vi "Main.vi"() -> ()   [LabVIEW 2024]
uses:
  <vilib>/userDefined/High Color/IMAQdx.ctl
  <vilib>/Utility/error.llb/DialogType.ctl
  <vilib>/addons/database/Connection.llb/Conn ObjectReference.ctl
  <vilib>/vision/Image Controls.llb/IMAQ Image.ctl
  <vilib>/vision/driver/IMAQdx.llb/IMAQdx Camera Control Mode.ctl
  <vilib>/addons/_JKI Toolkits/State Machine/_JKI_lib_State_Machine.llb/Select State(s)_err__jki_lib_state_machine.vi
  <vilib>/addons/_JKI Toolkits/State Machine/_JKI_lib_State_Machine.llb/Periodic Trigger__ogtk__JKI-SM__jki_lib_state_machine.vi
  <vilib>/addons/database/Auxilliary.llb/DB Tools Format Datetime String (Time Stamp).vi
  <vilib>/addons/database/NI_Database_API.lvlib
  <vilib>/vision/driver/NI_Vision_Acquisition_Software.lvlib
  <vilib>/addons/database/Connection.llb/DB Tools Open Connec (String).vi
panel:
  out "Error":bool
  out "Alarm":bool
  out "Measurement":dbl format="%#.2f"
  out "Database Save":bool
  out "Measuring":bool
  out "Is Measurement On":bool
  in  "Threshold":dbl(slide) min=0.0 max=100.0 step=5.0 scale=0.0..100.0
  in  "Source":bool
  in  "Camera":T1
  in  "Stop Application":bool
  in  "Stop Measurement":bool
  in  "Start Measurement":bool
  out "Image":T2(plugin-control)
  # "WLMS - Water Level Measuring\nSystem"
  # "Indicators"
  # "Is Measurement On"
  # "Currently Measuring"
  # "Saving To Database"
  # "Measurement Result, %"
  # "Alarm Level Detected"
  # "Error Occurred"
  # "Controls"
  # "Measurement Source"
  # "Camera"
  # "Image"
  # "Camera Source"
  # "Alarm Level Threshold"
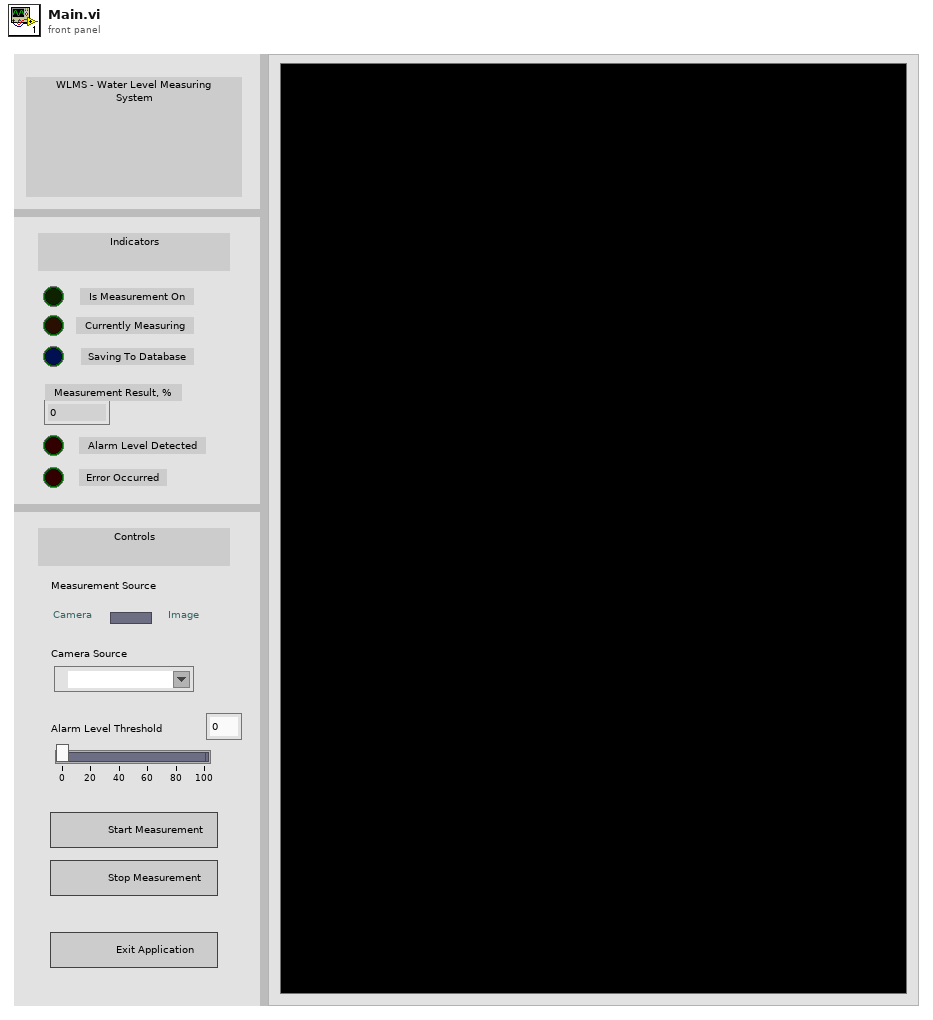
[diagram p1: front panel]
types:
  T1 = typedef "IMAQdx.ctl" = refnum<k21>
  T2 = typedef "IMAQ Image.ctl" = refnum<image>
  T3 = enum32{"Invalid", "Standard", "Closed", "Hidden", "Minimized", "Maximized"}
  T4 = enum32{"invalid app kind", "Development System", "Run Time System", "Student Edition", "Embedded LabVIEW", "Evaluation", "Custom"}
  T5 = typedef "NI_Vision_Acquisition_Software.lvlib/IMAQdx Camera Control Mode.ctl" = enum32{"Controller", "Listener"}
  T6 = typedef "NI_Database_API.lvlib/Conn ObjectReference.ctl" = refnum<k1>
  T7 = cluster{"Core":cluster{"Current VI Reference":refnum<vi>, "Close Panel on Exit?":bool}, "DB info":cluster{"DB connection":T6, "Table name":string, "Table columns":string[], "Connection string":string}, "Python info":cluster{"Function name":string, "Module name":string, "Python version":string, "Session reference":refnum<k35>}, "Measurement":cluster{"Is On":bool, "Period":u32, "Date":string, "Value":dbl, "Threshold":dbl, "Is Alarm On":bool, "LinePosY":i32}, "Camera data":cluster{"Camera":T1, "Image":T2, "Timeout":i32, "Frequency":i32, "Use image":bool, "Image name":string}}
  T8 = typedef "DialogType.ctl" = u16
  T9 = cluster{"Camera":T1, "Image":T2, "Timeout":i32, "Frequency":i32, "Use image":bool, "Image name":string}
  T10 = cluster{"Is On":bool, "Period":u32, "Date":string, "Value":dbl, "Threshold":dbl, "Is Alarm On":bool, "LinePosY":i32}
  T11 = cluster{"Function name":string, "Module name":string, "Python version":string, "Session reference":refnum<k35>}
  T12 = cluster{"DB connection":T6, "Table name":string, "Table columns":string[], "Connection string":string}
  T13 = cluster{"Current VI Reference":refnum<vi>, "Close Panel on Exit?":bool}
  T14 = cluster{"Desired Font (Application)":enum16{"User-specified Font", "Application Font", "System Font", "Dialog Font"}, "[User-specified Font]":cluster{"Font Name":string, "Size":i16, "Strikeout?":bool, "Italic?":bool, "Underline?":bool, "Outline?":bool, "Shadow?":bool, "Bold?":bool, "Rotation Angle":dbl}, "Horizontal Alignment":i16, "Vertical Alignment":i16}
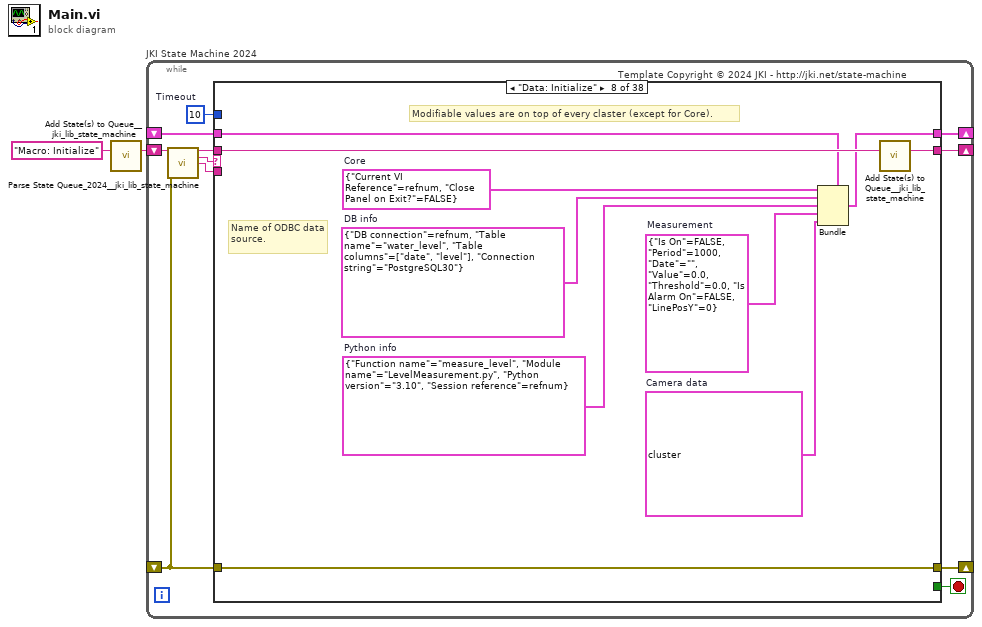
[diagram p0: block diagram]
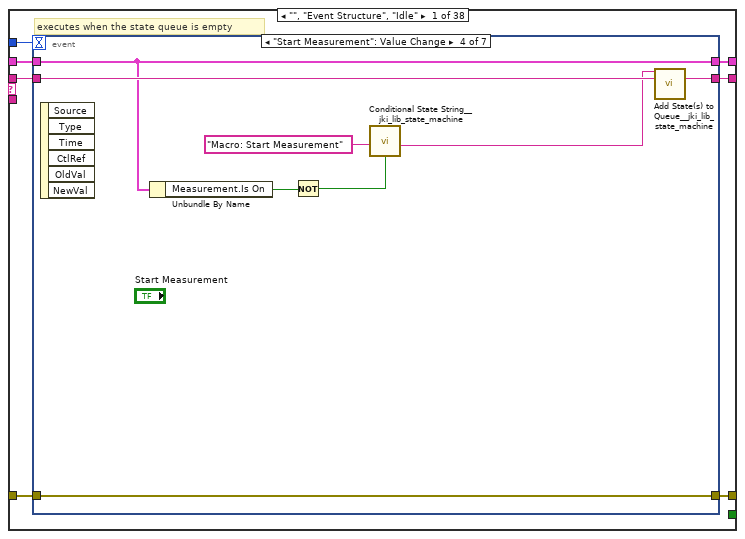
[diagram p2: hidden frame]
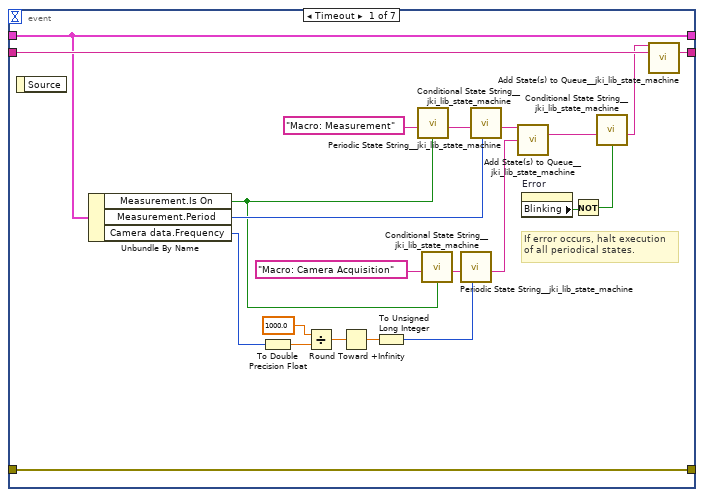
[diagram p3: hidden frame]
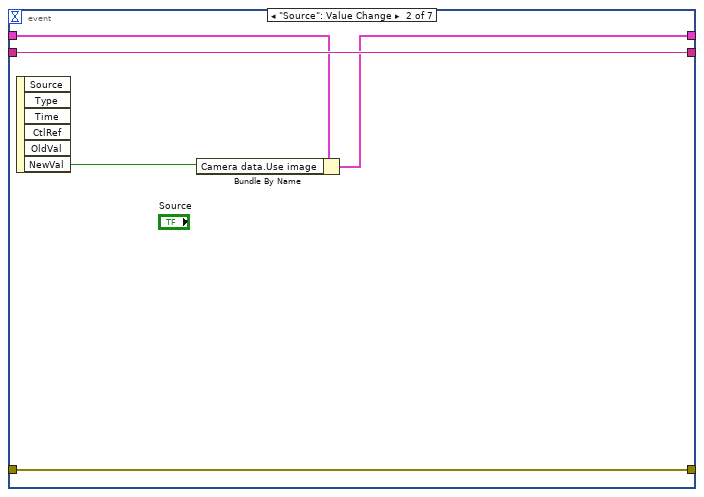
[diagram p4: hidden frame]
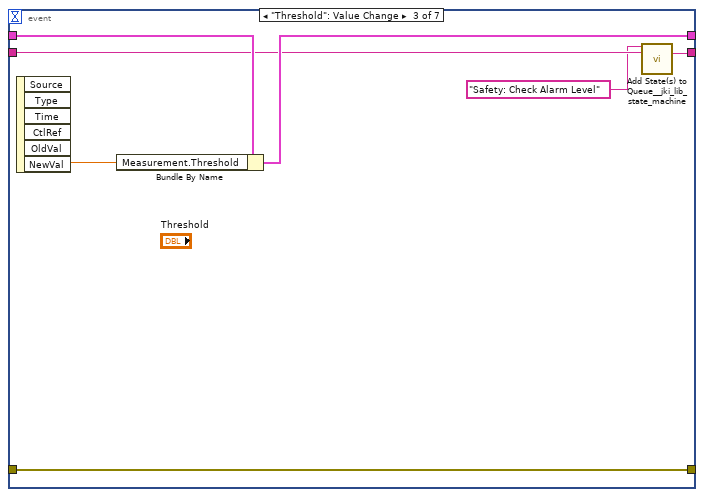
[diagram p5: hidden frame]
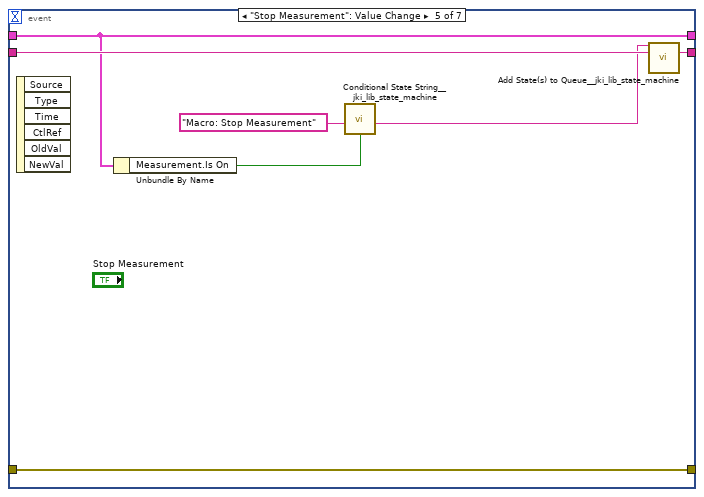
[diagram p6: hidden frame]
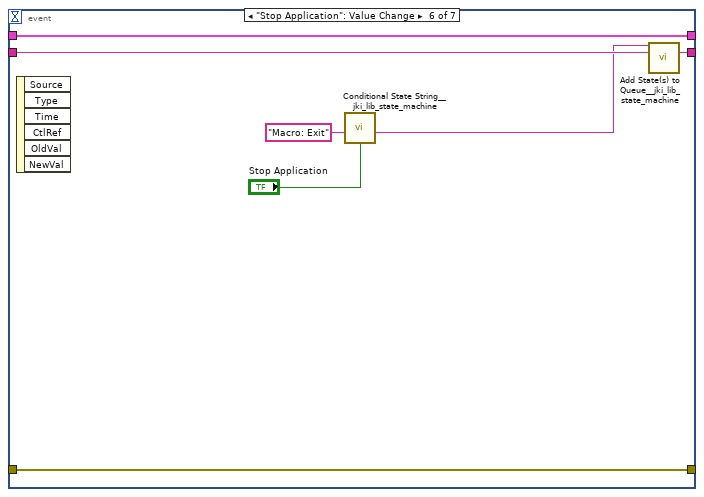
[diagram p7: hidden frame]
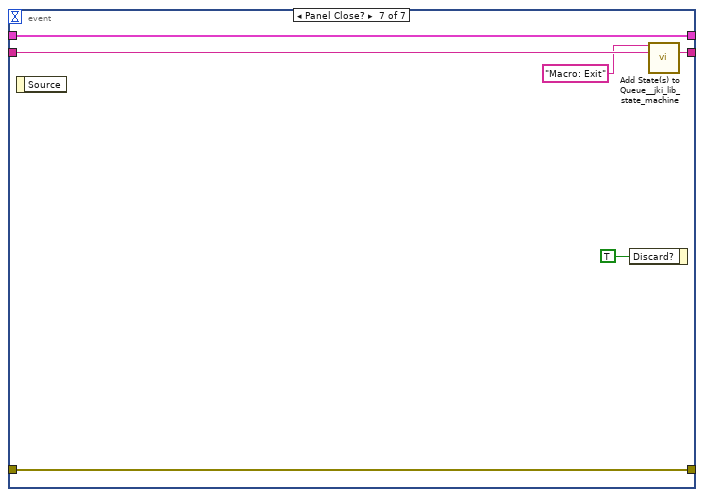
[diagram p8: hidden frame]
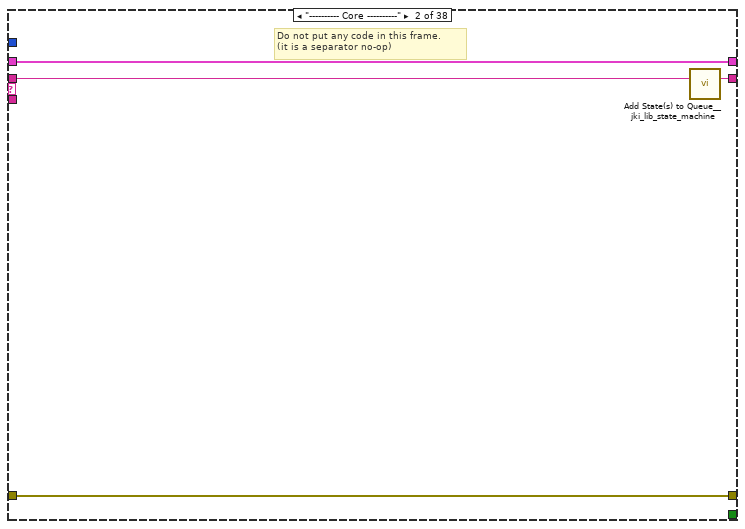
[diagram p9: hidden frame]
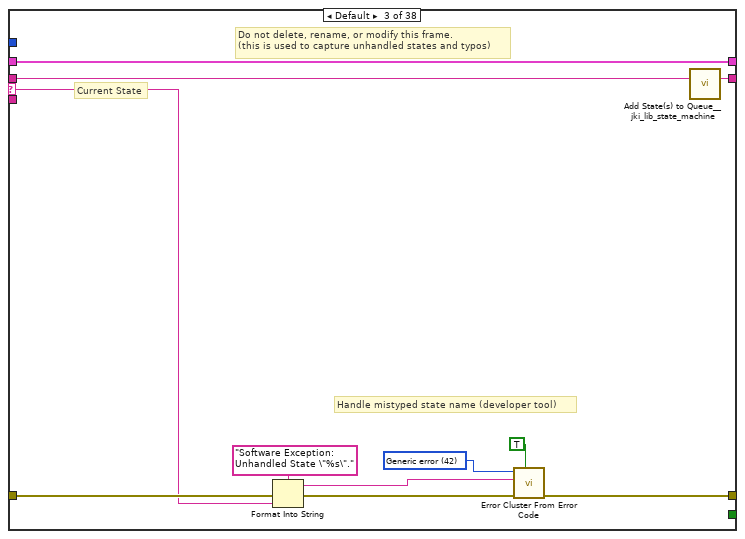
[diagram p10: hidden frame]
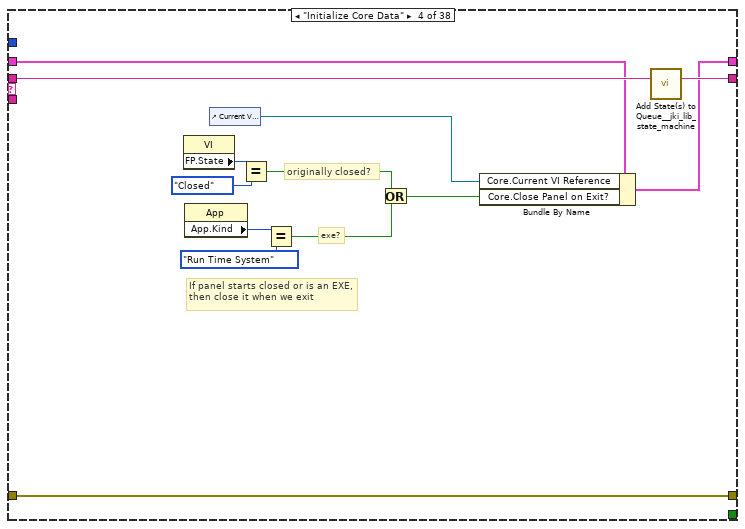
[diagram p11: hidden frame]
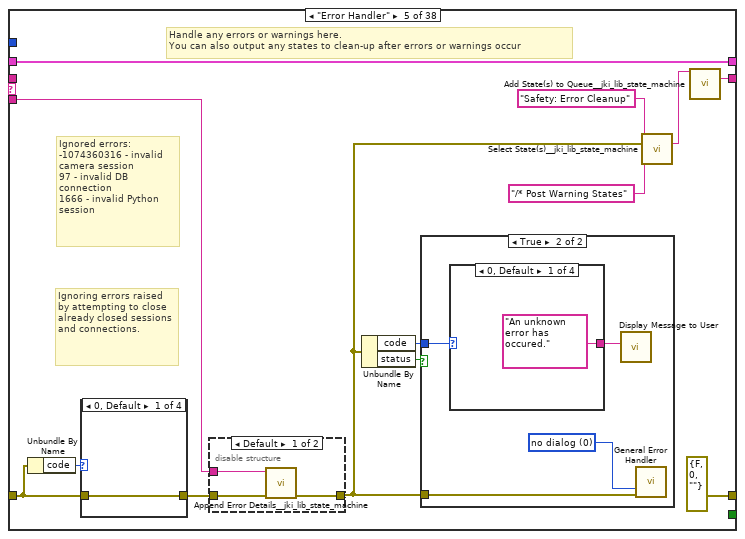
[diagram p12: hidden frame]
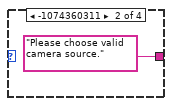
[diagram p14: hidden frame]
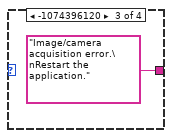
[diagram p15: hidden frame]
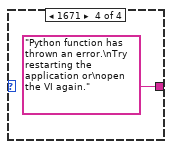
[diagram p16: hidden frame]
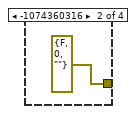
[diagram p17: hidden frame]
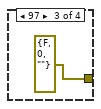
[diagram p18: hidden frame]
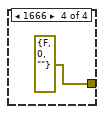
[diagram p19: hidden frame]
diagram:
  n1 = call <vilib>:"Add State(s) to Queue__jki_lib_state_machine.vi"("State(s) in (\"\")"="Macro: Initialize") -> ("States Out"=w2:string)  [unwired: 14 in]
  n2 = while "JKI State Machine 2024" {
    shift-right: [w7] -> _
    shift-left: _ -> [w6]
    shift-right: [w10] -> _
    shift-left: _ -> [w4]
    shift-right: [w9] -> _
    shift-left: w2 -> [w11]
    stop <- w8 stop-if-true
    w5 = 10  # Timeout
    # "Template Copyright © 2024 JKI - http://jki.net/state-machine"
    n3 = call <vilib>:"Parse State Queue_2024__jki_lib_state_machine.vi"("State Queue"=w11, "Error In (no error)"=w4) -> ("Remaining States"=w13:string, "Current State"=w3:string, "Arguments"=w12:string)  [unwired: 11 in]
    n4 = case shown="\"Data: Initialize\"" w3 {
      selector: w3 -> [_ _ w87 _ _ _ _ _ _ _ _ _ _ _ _ _ _ _ _ _ _ _ _ _ _ _ _ _ _ _ _ _ _ _ _ _ _ _]
      tunnel: w13 -> [w20 w86 w91 w110 _ w144 w148 w158 w164 w168 w179 w189 w195 w206 w270 w275 w283 w288 w295 w300 w312 w316 w324 w340 w346 w350 w364 w376 w421 w426 w432 w436 w444 w466 w472 w476 w485 w493]
      tunnel: w12 -> [_ _ _ _ w121 _ _ _ _ _ _ _ w190 w201 _ _ _ _ _ _ _ _ _ _ _ _ _ _ _ _ _ _ _ _ _ _ _ _]
      tunnel: w6 -> [w18 w83 w89 w98 w117 w142 w145 w149 w159 w165 w174 w181 w193 w200 w267 w272 w280 w284 w292 w297 w305 w313 w318 w333 w342 w347 w359 w374 w419 w422 w430 w433 w439 w456 w468 w473 w480 w488]
      tunnel: [w17 w84 w93 w108 errorcluster {"status"=FALSE, "code"=0, "source"=""} ("error out") w141 w146 w156 w161 w166 w177 w182 w191 w203 w268 w273 w278 w286 w290 w298 w308 w314 w319 w331 w343 w348 w351 w367 w399 w424 w427 w434 w440 w452 w469 w474 w483 w489] -> w10
      tunnel: w4 -> [w14 w84 w92 w108 w112 w141 w146 w156 w162 w166 w177 w183 w192 w204 w268 w273 w278 w286 w290 w298 w308 w314 w322 w337 w344 w348 w361 w371 w402 w424 w428 w434 w441 w464 w470 w474 w483 w489]
      tunnel: [w19 w85 w90 w109 w123 w143 w147 w157 w163 w167 w178 w188 w194 w205 w269 w274 w282 w287 w294 w299 w311 w315 w323 w339 w345 w349 w363 w375 w420 w425 w431 w435 w443 w465 w471 w475 w484 w492] -> w9
      tunnel: [_ _ _ _ _ TRUE _ _ _ _ _ _ _ _ _ _ _ _ _ _ _ _ _ _ _ _ _ _ _ _ _ _ _ _ _ _ _ _] -> w8
      tunnel: [w16 w83 w89 w99 w117 w142 w145 w152 w159 w165 w173 w181 w193 w200 w267 w272 w279 w284 w291 w297 w305 w313 w320 w333 w342 w347 w358 w373 w418 w422 w430 w433 w437 w455 w468 w473 w478 w487] -> w7
      tunnel: w5 -> [w15 _ _ _ _ _ _ _ _ _ _ _ _ _ _ _ _ _ _ _ _ _ _ _ _ _ _ _ _ _ _ _ _ _ _ _ _ _]
      frame "", "Event Structure", "Idle" {
        # "executes when the state queue is empty"
        n5 = event shown="[3] \"Start Measurement\": Value Change" {
          selector: _ -> [_ _ _ _ _ _ _]
          dyn-events: _ -> [_ _ _ _ _ _ _]
          timeout: w15 -> [_ _ _ _ _ _ _]
          tunnel: w20 -> [w42 w47 w49 w59 w69 w76 w82]
          tunnel: [w41 w47 w50 w60 w68 w75 w81] -> w19
          tunnel: w18 -> [w36 w46 w53 w57 w64 w73 w79]
          tunnel: [w40 w43 w54 w62 w67 w74 w80] -> w17
          tunnel: w14 -> [w40 w43 w54 w62 w67 w74 w80]
          tunnel: [w36 w44 w52 w57 w64 w73 w79] -> w16
          event Timeout {
            # "If error occurs, halt execution\nof all periodical states."
            n6 = event-data() -> ()  [unwired: 1 in, 1 out]
            n7 = Unbundle By Name(w36) -> ("Measurement.Is On"=w33:bool, "Measurement.Period"=w37:u32, "Camera data.Frequency"=w27:i32)
            n8 = To Double Precision Float(number=w27) -> (double precision float=w28:dbl)
            n9 = Divide(x=1000.0, y=w28) -> (x/y=w26:dbl)
            n10 = Round Toward +Infinity(x=w26) -> (ceil(x): smallest int >= x=w25:dbl)
            n11 = To Unsigned Long Integer(number=w25) -> (unsigned 32bit integer=w29:u32)
            n12 = call <vilib>:"Conditional State String__jki_lib_state_machine.vi"("Do State(s)?"=w33, "State"="Macro: Measurement") -> ("State Out"=w38:string)  [unwired: 7 in]
            n13 = call <vilib>:"Conditional State String__jki_lib_state_machine.vi"("Do State(s)?"=w33, "State"="Macro: Camera Acquisition") -> ("State Out"=w34:string)  [unwired: 7 in]
            n14 = call <vilib>:"Periodic State String__jki_lib_state_machine.vi"("Period (ms)"=w29, "State"=w34) -> ("State Out"=w31:string)  [unwired: 9 in]
            n15 = call <vilib>:"Periodic State String__jki_lib_state_machine.vi"("Period (ms)"=w37, "State"=w38) -> ("State Out"=w32:string)  [unwired: 9 in]
            n16 = call <vilib>:"Add State(s) to Queue__jki_lib_state_machine.vi"("State(s) in Front (\"\")"=w32, "State(s) at Back (\"\")"=w31) -> ("States Out"=w24:string)  [unwired: 13 in]
            n17 = property on="Error" class="Bool (strict)"() -> ("Blinking"=w22:bool)  [unwired: 2 in, 2 out]
            n18 = Not(x=w22) -> (.not. x?=w21:bool)
            n19 = call <vilib>:"Conditional State String__jki_lib_state_machine.vi"("Do State(s)?"=w21, "State"=w24) -> ("State Out"=w23:string)  [unwired: 7 in]
            n20 = call <vilib>:"Add State(s) to Queue__jki_lib_state_machine.vi"("State(s) in Front (\"\")"=w23, "State(s) in (\"\")"=w42) -> ("States Out"=w41:string)  [unwired: 13 in]
          }
          event "Source": Value Change {
            n21 = event-data() -> ("NewVal"=w45:bool)  [unwired: 1 in, 5 out]
            n22 = Bundle By Name(cluster=w46, "Camera data.Use image"=w45) -> (w44:T7)
          }
          event "Threshold": Value Change {
            n23 = event-data() -> ("NewVal"=w51:dbl)  [unwired: 1 in, 5 out]
            n24 = Bundle By Name(cluster=w53, "Measurement.Threshold"=w51) -> (w52:T7)
            n25 = call <vilib>:"Add State(s) to Queue__jki_lib_state_machine.vi"("State(s) in Front (\"\")"="Safety: Check Alarm Level", "State(s) in (\"\")"=w49) -> ("States Out"=w50:string)  [unwired: 13 in]
          }
          event "Start Measurement": Value Change {
            n26 = event-data() -> ()  [unwired: 1 in, 6 out]
            n27 = Unbundle By Name(w57) -> ("Measurement.Is On"=w56:bool)
            n28 = Not(x=w56) -> (.not. x?=w55:bool)
            n29 = call <vilib>:"Conditional State String__jki_lib_state_machine.vi"("Do State(s)?"=w55, "State"="Macro: Start Measurement") -> ("State Out"=w58:string)  [unwired: 7 in]
            n30 = call <vilib>:"Add State(s) to Queue__jki_lib_state_machine.vi"("State(s) in Front (\"\")"=w58, "State(s) in (\"\")"=w59) -> ("States Out"=w60:string)  [unwired: 13 in]
          }
          event "Stop Measurement": Value Change {
            n31 = event-data() -> ()  [unwired: 1 in, 6 out]
            n32 = Unbundle By Name(w64) -> ("Measurement.Is On"=w63:bool)
            n33 = call <vilib>:"Conditional State String__jki_lib_state_machine.vi"("Do State(s)?"=w63, "State"="Macro: Stop Measurement") -> ("State Out"=w65:string)  [unwired: 7 in]
            n34 = call <vilib>:"Add State(s) to Queue__jki_lib_state_machine.vi"("State(s) in Front (\"\")"=w65, "State(s) in (\"\")"=w69) -> ("States Out"=w68:string)  [unwired: 13 in]
          }
          event "Stop Application": Value Change {
            n35 = event-data() -> ()  [unwired: 1 in, 6 out]
            n36 = call <vilib>:"Conditional State String__jki_lib_state_machine.vi"("Do State(s)?"="Stop Application", "State"="Macro: Exit") -> ("State Out"=w71:string)  [unwired: 7 in]
            n37 = call <vilib>:"Add State(s) to Queue__jki_lib_state_machine.vi"("State(s) in Front (\"\")"=w71, "State(s) in (\"\")"=w76) -> ("States Out"=w75:string)  [unwired: 13 in]
          }
          event Panel Close? {
            n38 = event-data() -> ()  [unwired: 1 in, 1 out]
            n39 = event-data("Discard?"=TRUE) -> ()  [unwired: 1 in, 1 out]
            n40 = call <vilib>:"Add State(s) to Queue__jki_lib_state_machine.vi"("State(s) in Front (\"\")"="Macro: Exit", "State(s) in (\"\")"=w82) -> ("States Out"=w81:string)  [unwired: 13 in]
          }
        }
      }
      frame "---------- Core ----------" {
        # "Do not put any code in this frame.\n(it is a separator no-op)"
        n41 = call <vilib>:"Add State(s) to Queue__jki_lib_state_machine.vi"("State(s) in (\"\")"=w86) -> ("States Out"=w85:string)  [unwired: 14 in]
      }
      frame Default {
        w96 = 42 items=["No error", "Argument error", "Memory is full", "Out of zone", "End of file", "File already open", "Generic file I/O error", "File not found", "File permission error", "Disk is full", "Duplicate path", "Too many files open", "System feature not enabled", "Resource file not found", "Cannot add resource", "Resource not found", "Image not found", "Image memory error", "Pen does not exist", "Config type invalid", "Config token not found", "Config parse error", "Config memory error", "Bad external code format", "Bad external code offset", "External code not present", "Null window", "Destroy window error", "Null menu", "Print aborted", "Bad print record", "Print driver error", "Windows error during printing", "Memory error during printing", "Print dialog error", "Generic print error", "Invalid device refnum", "Device not found", "Device parameter error", "Device unit error", "Cannot open device", "Device call aborted", "Generic error", "Cancelled by user", "Object ID too low", "Object ID too high", "Object not in heap", "Unknown heap", "Unknown object (invalid DefProc)", "Unknown object (DefProc not in table)", "Message out of range", "Invalid (null) method", "Unknown message", "Manager call not supported", "Bad address", "Network operation in progress", "Network operation timed out", "Connection is busy", "Network attribute not supported", "Network error", "Address in use", "System out of memory", "Connection aborted", "Connection refused", "Not connected", "Already connected", "Connection closed", "Initialization error (interapplication manager)", "Bad occurrence", "Wait on unbound occurrence handler", "Occurrence queue overflow", "Datalog type conflict", "Unused", "Unrecognized type (interapplication manager)", "Memory corrupt", "Failed to make temporary DLL", "Old CIN version", "Drag socket not found", "Failed to load drop-object", "Failed to register OLE object", "Failed to release OLE object", "Format specifier type mismatch", "Unknown format specifier", "Too few format specifiers", "Too many format specifiers", "Scan failed", "Newer CIN version", "Error converting to variant", "Runtime menu error", "Password tampered", "Variant attribute not found", "Incompatible variant data type", "Event data is not available", "Event Store is not present", "Occurrence is not found", "Event Queue is not created", "Event info is not available", "Refnum passed is NULL", "Error retrieving Class GUID", "Error retrieving CoClass GUID", "Error retrieving TypeLib GUID.", "Bad built application magic bytes.", "Specific driver is different from the specific driver associated with the Logical Name.", "There is no session opened to the class driver.", "Max Error", "MAX - Error with config objects", "MAX - Error loading configuration", "MAX - Group not supported"]
        # "Current State"
        # "Do not delete, rename, or modify this frame.\n(this is used to capture unhandled states and typos)"
        # "Handle mistyped state name (developer tool)"
        n42 = Format Into String(format string="Software Exception: Unhandled State \"%s\"." ("message"), error in=w92, w87) -> (resulting string=w95:string, error out=w94:errorcluster)  [unwired: 1 in]
        n43 = call <vilib>:"Error Cluster From Error Code.vi"("show call chain? (False)"=TRUE, "error in (no error)"=w94, "error message (\"\")"=w95, "error code (0)"=w96) -> ("error out"=w93:errorcluster)  [unwired: 5 in]
        n44 = call <vilib>:"Add State(s) to Queue__jki_lib_state_machine.vi"("State(s) in (\"\")"=w91) -> ("States Out"=w90:string)  [unwired: 14 in]
      }
      frame "Initialize Core Data" {
        # "originally closed?"
        # "exe?"
        # "If panel starts closed or is an EXE, then close it when we exit"
        n45 = property class="VI"() -> ("FP.State"=w102:T3)  [unwired: 2 in, 2 out]
        n46 = property class="App"() -> ("App.Kind"=w107:T4)  [unwired: 2 in, 2 out]
        n47 = control-ref of="Current VI Reference"() -> (w103:refnum<vi>)
        n48 = Equal?(x=w102, y=T3."Closed" ("Front Panel Window:State")) -> (x = y?=w100:bool)
        n49 = Equal?(x=w107, y=T4."Run Time System" ("Application:Kind")) -> (x = y?=w105:bool)
        n50 = Or(x=w100, y=w105) -> (x .or. y?=w104:bool)
        n51 = Bundle By Name(cluster=w98, "Core.Current VI Reference"=w103, "Core.Close Panel on Exit?"=w104) -> (w99:T7)
        n52 = call <vilib>:"Add State(s) to Queue__jki_lib_state_machine.vi"("State(s) in (\"\")"=w110) -> ("States Out"=w109:string)  [unwired: 14 in]
      }
      frame "Error Handler" {
        # "Ignored errors:\n-1074360316 - invalid\ncamera session\n97 - invalid DB connection\n1666 - invalid Python session"
        # "Ignoring errors raised by attempting to close already closed sessions and connections."
        # "Handle any errors or warnings here.\nYou can also output any states to clean-up after errors or warnings occur"
        n53 = Unbundle By Name(w112) -> ("code"=w114:i32)
        n54 = case shown="0, Default" w114 {
          tunnel: [w132 errorcluster {"status"=FALSE, "code"=0, "source"=""} ("error out") errorcluster {"status"=FALSE, "code"=0, "source"=""} ("error out") errorcluster {"status"=FALSE, "code"=0, "source"=""} ("error out")] -> w113
          tunnel: w112 -> [w132 _ _ _]
          frame 0, Default {
          }
          frame -1074360316 {
          }
          frame 97 {
          }
          frame 1666 {
          }
        }
        n55 = disable-structure shown="Default" {
          disable-tunnel: w113 -> [w138 w139]
          disable-tunnel: w121 -> [w137 _]
          disable-tunnel: [w136 w139] -> w115
          frame condition #0 (active) {
            n56 = call <vilib>:"Append Error Details__jki_lib_state_machine.vi"("error in (no error)"=w138, "Previous State and Argument(s)"=w137) -> ("error out"=w136:errorcluster)  [unwired: 9 in]
          }
          frame condition #1 {
          }
        }
        n57 = Unbundle By Name(w115) -> ("code"=w116:i32, "status"=w111:bool)
        n58 = case shown="True" w111 {
          tunnel: w116 -> [_ w126]
          tunnel: w115 -> [_ w125]
          frame False {
          }
          frame True {
            w124 = T8 0 items=["no dialog", "OK message", "continue or stop message", "OK message + warnings", "continue/stop + warnings"] ("type of dialog (OK msg:1)")
            n59 = case shown="0, Default" w126 {
              tunnel: ["An unknown error has occured." "Please choose valid camera source." "Image/camera acquisition error.\nRestart the application." "Python function has thrown an error.\nTry restarting the application or\nopen the VI again."] -> w127
              frame 0, Default {
              }
              frame -1074360311 {
              }
              frame -1074396120 {
              }
              frame 1671 {
              }
            }
            n60 = call "Display Message to User"("Message"=w127) -> ()  [unwired: 9 in, 2 out]
            n61 = call <vilib>:"General Error Handler.vi"("type of dialog (OK msg:1)"=w124, "error in (no error)"=w125) -> ()  [unwired: 9 in, 5 out]
          }
        }
        n62 = call-poly <vilib>:"Select State(s)__jki_lib_state_machine.vi"("State(s) if True (\"\")"="Safety: Error Cleanup", "Select"=w115, "State(s) if False (\"\")"="/* Post Warning States") -> ("States Out"=w119:string)  [unwired: 12 in]
        n63 = call <vilib>:"Add State(s) to Queue__jki_lib_state_machine.vi"("State(s) in Front (\"\")"=w119) -> ("States Out"=w123:string)  [unwired: 14 in]
      }
      frame "Exit" {
        # "Do not put any code in this frame.\n(No errors that occur here will be handled.)"
        n64 = call <vilib>:"Add State(s) to Queue__jki_lib_state_machine.vi"("State(s) in (\"\")"=w144) -> ("States Out"=w143:string)  [unwired: 14 in]
      }
      frame "---------- Data ----------" {
        # "Do not put any code in this frame.\n(It is a separator no-op. You can make a copy of this frame to create a new Data frame)"
        n65 = call <vilib>:"Add State(s) to Queue__jki_lib_state_machine.vi"("State(s) in (\"\")"=w148) -> ("States Out"=w147:string)  [unwired: 14 in]
      }
      frame "Data: Initialize" {
        w150 = T9 {"Camera"="", "Image"=refnum, "Timeout"=5000, "Frequency"=25, "Use image"=TRUE, "Image name"="firstframe.jpg"}  # Camera data
        w151 = T10 {"Is On"=FALSE, "Period"=1000, "Date"="", "Value"=0.0, "Threshold"=0.0, "Is Alarm On"=FALSE, "LinePosY"=0}  # Measurement
        w153 = T11 {"Function name"="measure_level", "Module name"="LevelMeasurement.py", "Python version"="3.10", "Session reference"=refnum}  # Python info
        w154 = T12 {"DB connection"=refnum, "Table name"="water_level", "Table columns"=["date", "level"], "Connection string"="PostgreSQL30"}  # DB info
        w155 = T13 {"Current VI Reference"=refnum, "Close Panel on Exit?"=FALSE}  # Core
        # "Modifiable values are on top of every claster (except for Core)."
        # "Name of ODBC data source."
        n66 = Bundle(cluster=w149, "Core"=w155, "DB info"=w154, "Python info"=w153, "Measurement"=w151, "Camera data"=w150) -> (w152:T7)
        n67 = call <vilib>:"Add State(s) to Queue__jki_lib_state_machine.vi"("State(s) in (\"\")"=w158) -> ("States Out"=w157:string)  [unwired: 14 in]
      }
      frame "Data: Cleanup" {
        n68 = Unbundle By Name(w159) -> ("Core.Current VI Reference"=w160:refnum<vi>)
        n69 = Close Reference(reference=w160, error in (no error)=w162) -> (error out=w161:errorcluster)
        n70 = call <vilib>:"Add State(s) to Queue__jki_lib_state_machine.vi"("State(s) in (\"\")"=w164) -> ("States Out"=w163:string)  [unwired: 14 in]
      }
      frame "---------- UI ----------" {
        # "Do not put any code in this frame.\n(It is a separator no-op. You can make a copy of this frame to create a new UI frame)"
        n71 = call <vilib>:"Add State(s) to Queue__jki_lib_state_machine.vi"("State(s) in (\"\")"=w168) -> ("States Out"=w167:string)  [unwired: 14 in]
      }
      frame "UI: Initialize" {
        w171 = FALSE ("Database Save")
        n72 = property on="Source" class="Bool (strict)"() -> ("Value"=w175:bool)  [unwired: 2 in, 2 out]
        n73 = property on="Threshold" class="Slide (strict)"() -> ("Value"=w172:dbl)  [unwired: 2 in, 2 out]
        n74 = Bundle By Name(cluster=w174, "Camera data.Use image"=w175, "Measurement.Threshold"=w172) -> (w173:T7)
        n75 = property on="Is Measurement On" class="Bool (strict)"("Value"=w171) -> ()  [unwired: 2 in, 2 out]
        n76 = property on="Database Save" class="Bool (strict)"("Value"=w171) -> ()  [unwired: 2 in, 2 out]
        n77 = property on="Measuring" class="Bool (strict)"("Value"=w171) -> ()  [unwired: 2 in, 2 out]
        n78 = property on="Measurement" class="DigNum (strict)"("Value"=0.0 ("Measurement")) -> ()  [unwired: 2 in, 2 out]
        n79 = property on="Alarm" class="Bool (strict)"("Blinking"=FALSE) -> ()  [unwired: 2 in, 2 out]
        n80 = property on="Error" class="Bool (strict)"("Blinking"=FALSE) -> ()  [unwired: 2 in, 2 out]
        n81 = call <vilib>:"Add State(s) to Queue__jki_lib_state_machine.vi"("State(s) in (\"\")"=w179) -> ("States Out"=w178:string)  [unwired: 14 in]
      }
      frame "UI: Uninitialize" {
        w187 = FALSE ("Database Save")
        w185 = T2 refnum  # Image
        n82 = To Variant(anything=w185) -> (Variant=w184:variant)
        n83 = property on="Measuring" class="Bool (strict)"("Value"=w187) -> ()  [unwired: 2 in, 2 out]
        n84 = property on="Is Measurement On" class="Bool (strict)"("Value"=w187) -> ()  [unwired: 2 in, 2 out]
        n85 = property on="Database Save" class="Bool (strict)"("Value"=w187) -> ()  [unwired: 2 in, 2 out]
        n86 = property on="Measurement" class="DigNum (strict)"("Value"=0.0 ("Measurement")) -> ()  [unwired: 2 in, 2 out]
        n87 = property on="Image" class="ImageControl"("Value"=w184) -> ()  [unwired: 2 in, 2 out]
        n88 = Unbundle By Name(w181) -> ("Camera data.Image"=w180:T2)
        n89 = call "IMAQ Dispose"("Image"=w180, "error in (no error)"=w183) -> ("error out"=w182:errorcluster)  [unwired: 4 in]
        n90 = call <vilib>:"Add State(s) to Queue__jki_lib_state_machine.vi"("State(s) in (\"\")"=w189) -> ("States Out"=w188:string)  [unwired: 14 in]
      }
      frame "UI: Cursor Set" {
        # "Argument"
        n91 = case shown="\"Busy\"" w190 {
          tunnel: w192 -> [w197 w199]
          tunnel: [w196 w198] -> w191
          frame "Idle", Default {
            n92 = call <vilib>:"Unset Busy.vi"("error in (no error)"=w197) -> ("error out"=w196:errorcluster)  [unwired: 10 in]
          }
          frame "Busy" {
            n93 = call <vilib>:"Set Busy.vi"("error in (no error)"=w199) -> ("error out"=w198:errorcluster)  [unwired: 9 in, 1 out]
          }
        }
        n94 = call <vilib>:"Add State(s) to Queue__jki_lib_state_machine.vi"("State(s) in (\"\")"=w195) -> ("States Out"=w194:string)  [unwired: 14 in]
      }
      frame "UI: Front Panel State" {
        # "Argument"
        n95 = Unbundle By Name(w200) -> ("Core.Current VI Reference"=w202:refnum<vi>)
        n96 = case shown="\"Open\", \"Standard\", Default" w201 {
          tunnel: w204 -> [w212 w225 w236 w248 w260]
          tunnel: [w213 w226 w237 w249 w261] -> w203
          tunnel: w202 -> [_ _ _ _ _]
          frame "Open", "Standard", Default {
            w207 = T3."Standard" ("State")
            n97 = property class="VI"(error in=w212) -> (reference out=w210:refnum<vi>, error out=w211:errorcluster, "FP.State"=w209:T3)  [unwired: 1 in]
            n98 = Not Equal?(x=w209, y=w207) -> (x != y?=w208:bool)
            n99 = case shown="True" w208 {
              tunnel: [w217 w219] -> w213
              tunnel: w211 -> [w216 w219]
              tunnel: w210 -> [w215 _]
              tunnel: w207 -> [w214 _]
              frame True {
                n100 = invoke class="VI" method="FP.Open"(reference=w215, error in=w216, "Activate"=TRUE, "State"=w214) -> (error out=w217:errorcluster)  [unwired: 1 in, 4 out]
              }
              frame False {
              }
            }
          }
          frame "Close", "Closed" {
            n101 = property class="VI"(error in=w225) -> (reference out=w223:refnum<vi>, error out=w224:errorcluster, "FP.State"=w221:T3)  [unwired: 1 in]
            n102 = Not Equal?(x=w221, y=T3."Closed" ("Front Panel Window:State")) -> (x != y?=w220:bool)
            n103 = case shown="True" w220 {
              tunnel: [w227 w230] -> w226
              tunnel: w224 -> [w227 w229]
              tunnel: w223 -> [_ w228]
              frame False {
              }
              frame True {
                n104 = invoke class="VI" method="FP.Close"(reference=w228, error in=w229) -> (error out=w230:errorcluster)  [unwired: 1 in, 2 out]
              }
            }
          }
          frame "Hidden", "Hide" {
            w231 = T3."Hidden" ("State")
            n105 = property class="VI"(error in=w236) -> (reference out=w234:refnum<vi>, error out=w235:errorcluster, "FP.State"=w233:T3)  [unwired: 1 in]
            n106 = Not Equal?(x=w233, y=w231) -> (x != y?=w232:bool)
            n107 = case shown="True" w232 {
              tunnel: [w241 w242] -> w237
              tunnel: w235 -> [w240 w242]
              tunnel: w234 -> [w239 _]
              tunnel: w231 -> [w238 _]
              frame True {
                n108 = invoke class="VI" method="FP.Open"(reference=w239, error in=w240, "State"=w238) -> (error out=w241:errorcluster)  [unwired: 2 in, 4 out]
              }
              frame False {
              }
            }
          }
          frame "Minimize", "Minimized" {
            w243 = T3."Minimized" ("State")
            n109 = property class="VI"(error in=w248) -> (reference out=w246:refnum<vi>, error out=w247:errorcluster, "FP.State"=w245:T3)  [unwired: 1 in]
            n110 = Not Equal?(x=w245, y=w243) -> (x != y?=w244:bool)
            n111 = case shown="True" w244 {
              tunnel: [w253 w254] -> w249
              tunnel: w247 -> [w252 w254]
              tunnel: w246 -> [w251 _]
              tunnel: w243 -> [w250 _]
              frame True {
                n112 = invoke class="VI" method="FP.Open"(reference=w251, error in=w252, "State"=w250) -> (error out=w253:errorcluster)  [unwired: 2 in, 4 out]
              }
              frame False {
              }
            }
          }
          frame "Maximize", "Maximized" {
            w255 = T3."Maximized" ("State")
            n113 = property class="VI"(error in=w260) -> (reference out=w258:refnum<vi>, error out=w259:errorcluster, "FP.State"=w257:T3)  [unwired: 1 in]
            n114 = Not Equal?(x=w257, y=w255) -> (x != y?=w256:bool)
            n115 = case shown="True" w256 {
              tunnel: [w265 w266] -> w261
              tunnel: w259 -> [w264 w266]
              tunnel: w258 -> [w263 _]
              tunnel: w255 -> [w262 _]
              frame True {
                n116 = invoke class="VI" method="FP.Open"(reference=w263, error in=w264, "State"=w262) -> (error out=w265:errorcluster)  [unwired: 2 in, 4 out]
              }
              frame False {
              }
            }
          }
        }
        n117 = call <vilib>:"Add State(s) to Queue__jki_lib_state_machine.vi"("State(s) in (\"\")"=w206) -> ("States Out"=w205:string)  [unwired: 14 in]
      }
      frame "---------- Macro ----------" {
        # "Do not put any code in this frame.\n(It is a separator no-op. You can make a copy of this frame to create a new Macro frame)"
        n118 = call <vilib>:"Add State(s) to Queue__jki_lib_state_machine.vi"("State(s) in (\"\")"=w270) -> ("States Out"=w269:string)  [unwired: 14 in]
      }
      frame "Macro: Initialize" {
        w271 = "Data: Initialize\nInitialize Core Data\nUI: Initialize\nUI: Front Panel State >> Open"  # Data: Initialize Initialize Core Data UI: Initialize UI: Front Panel State >> Open
        n119 = call <vilib>:"Add State(s) to Queue__jki_lib_state_machine.vi"("State(s) in Front (\"\")"=w271, "State(s) in (\"\")"=w275) -> ("States Out"=w274:string)  [unwired: 13 in]
      }
      frame "Macro: Start Measurement" {
        w277 = TRUE ("Measurement.Is On")
        n120 = property on="Error" class="Bool (strict)"("Blinking"=FALSE) -> ()  [unwired: 2 in, 2 out]
        n121 = Bundle By Name(cluster=w280, "Measurement.Is On"=w277) -> (w279:T7)
        n122 = property on="Is Measurement On" class="Bool (strict)"("Value"=w277) -> ()  [unwired: 2 in, 2 out]
        n123 = call <vilib>:"Add State(s) to Queue__jki_lib_state_machine.vi"("State(s) in Front (\"\")"="Camera: Initialize\nDatabase: Connect\nPython: Open Session", "State(s) in (\"\")"=w283) -> ("States Out"=w282:string)  [unwired: 13 in]
      }
      frame "Macro: Measurement" {
        n124 = call <vilib>:"Add State(s) to Queue__jki_lib_state_machine.vi"("State(s) in Front (\"\")"="Python: Fetch Level\nSafety: Check Alarm Level\nDatabase: Save Data" ("State(s) in Front (\"\")"), "State(s) in (\"\")"=w288) -> ("States Out"=w287:string)  [unwired: 13 in]
      }
      frame "Macro: Stop Measurement" {
        w289 = FALSE ("Measurement.Is On")
        n125 = Bundle By Name(cluster=w292, "Measurement.Is On"=w289) -> (w291:T7)
        n126 = property on="Is Measurement On" class="Bool (strict)"("Value"=w289) -> ()  [unwired: 2 in, 2 out]
        n127 = call <vilib>:"Add State(s) to Queue__jki_lib_state_machine.vi"("State(s) in Front (\"\")"="Camera: Remove\nDatabase: Disconnect \nPython: Close Session", "State(s) in (\"\")"=w295) -> ("States Out"=w294:string)  [unwired: 13 in]
      }
      frame "Macro: Camera Acquisition" {
        n128 = call <vilib>:"Add State(s) to Queue__jki_lib_state_machine.vi"("State(s) in Front (\"\")"="Camera: Read\nCamera: Add Data\nCamera: Display" ("State(s) in Front (\"\")"), "State(s) in (\"\")"=w300) -> ("States Out"=w299:string)  [unwired: 13 in]
      }
      frame "Macro: Exit" {
        n129 = Unbundle By Name(w305) -> ("Core.Close Panel on Exit?"=w306:bool, "Measurement.Is On"=w303:bool)
        n130 = call <vilib>:"Conditional State String__jki_lib_state_machine.vi"("Do State(s)?"=w306, "State"="UI: Front Panel State >> Close") -> ("State Out"=w304:string)  [unwired: 7 in]
        n131 = call <vilib>:"Conditional State String__jki_lib_state_machine.vi"("Do State(s)?"=w303, "State"="Macro: Stop Measurement") -> ("State Out"=w301:string)  [unwired: 7 in]
        n132 = call <vilib>:"Add State(s) to Queue__jki_lib_state_machine.vi"("State(s) in Front (\"\")"=w304, "State(s) in (\"\")"=w301, "State(s) at Back (\"\")"="UI: Uninitialize\nData: Cleanup\nExit") -> ("States Out"=w309:string)  [unwired: 12 in]
        n133 = call <vilib>:"Add State(s) to Queue__jki_lib_state_machine.vi"("State(s) in Front (\"\")"=w309, "State(s) in (\"\")"=w312) -> ("States Out"=w311:string)  [unwired: 13 in]
      }
      frame "---------- Database ----------" {
        # "Do not put any code in this frame.\n(It is a separator no-op. You can make a copy of this frame to create a new Macro frame)"
        n134 = call <vilib>:"Add State(s) to Queue__jki_lib_state_machine.vi"("State(s) in (\"\")"=w316) -> ("States Out"=w315:string)  [unwired: 14 in]
      }
      frame "Database: Connect" {
        n135 = Unbundle By Name(w318) -> ("DB info.Connection string"=w317:string)
        n136 = call-poly <vilib>:"DB Tools Open Connection.vi"("error in (no error)"=w322, "connection information"=w317) -> ("error out"=w319:errorcluster, "connection reference"=w321:T6)  [unwired: 6 in]
        n137 = Bundle By Name(cluster=w318, "DB info.DB connection"=w321) -> (w320:T7)
        n138 = call <vilib>:"Add State(s) to Queue__jki_lib_state_machine.vi"("State(s) in (\"\")"=w324) -> ("States Out"=w323:string)  [unwired: 14 in]
      }
      frame "Database: Save Data" {
        # "Jeżeli nie ma błędu, status przyjmuje wartość false. Jest to wykorzystane do sterowania kontrolką informującą o trwającym zapisie do bazy danych."
        n139 = Unbundle By Name(w333) -> ("Measurement.Date"=w326:string, "Measurement.Value"=w327:dbl, "DB info.DB connection"=w334:T6, "DB info.Table name"=w336:string, "DB info.Table columns"=w335:string[])
        n140 = Bundle(cluster=cluster{string, dbl} {"", 0.0}, w326, w327) -> (w328:cluster{string, dbl})
        n141 = To Variant(anything=w328) -> (Variant=w325:variant)
        n142 = call <vilib>:"DB Tools Insert Data.vi"("create table? (F)"=TRUE, "data"=w325, "error in (no error)"=w337, "columns"=w335, "table"=w336, "connection reference"=w334) -> ("error out"=w331:errorcluster)  [unwired: 4 in, 1 out]
        n143 = Unbundle By Name(w331) -> ("status"=w330:bool)
        n144 = property on="Database Save" class="Bool (strict)"("Value"=w330) -> ()  [unwired: 2 in, 2 out]
        n145 = call <vilib>:"Add State(s) to Queue__jki_lib_state_machine.vi"("State(s) in (\"\")"=w340) -> ("States Out"=w339:string)  [unwired: 14 in]
        "Database Save" <- TRUE ("Database Save")
      }
      frame "Database: Disconnect" {
        n146 = Unbundle By Name(w342) -> ("DB info.DB connection"=w341:T6)
        n147 = call <vilib>:"DB Tools Close Connection.vi"("error in (no error)"=w344, "connection reference"=w341) -> ("error out"=w343:errorcluster)  [unwired: 5 in]
        n148 = call <vilib>:"Add State(s) to Queue__jki_lib_state_machine.vi"("State(s) in (\"\")"=w346) -> ("States Out"=w345:string)  [unwired: 14 in]
      }
      frame "---------- Camera ----------" {
        # "Do not put any code in this frame.\n(It is a separator no-op. You can make a copy of this frame to create a new Macro frame)"
        n149 = call <vilib>:"Add State(s) to Queue__jki_lib_state_machine.vi"("State(s) in (\"\")"=w350) -> ("States Out"=w349:string)  [unwired: 14 in]
      }
      frame "Camera: Initialize" {
        n150 = call <vilib>:"IMAQdx Open Camera.vi"("Camera Control Mode"=IMAQdx_Camera_Control_Mode."Controller", "error in"=w361, "Session In"="Camera") -> ("error out"=w357:errorcluster, "Session Out"=w356:T1)  [unwired: 7 in]
        n151 = call <vilib>:"IMAQdx Configure Grab.vi"("error in"=w357, "Session In"=w356) -> ("error out"=w353:errorcluster, "Session Out"=w355:T1)  [unwired: 8 in]
        n152 = call "IMAQ Create"("Image Name"="Measurement", "error in (no error)"=w353) -> ("New Image"=w352:T2, "error out"=w351:errorcluster)  [unwired: 3 in]
        n153 = Bundle By Name(cluster=w359, "Camera data.Camera"=w355, "Camera data.Image"=w352) -> (w358:T7)
        n154 = call <vilib>:"Add State(s) to Queue__jki_lib_state_machine.vi"("State(s) in (\"\")"=w364) -> ("States Out"=w363:string)  [unwired: 14 in]
      }
      frame "Camera: Read" {
        n155 = Unbundle By Name(w374) -> ("Camera data.Use image"=w366:bool, "Camera data.Timeout"=w372:i32, "Camera data.Camera"=w369:T1, "Camera data.Image"=w370:T2, "Camera data.Image name"=w365:string)
        n156 = case shown="True" w366 {
          tunnel: w372 -> [w382 _]
          tunnel: w371 -> [w381 w385]
          tunnel: w370 -> [w377 w386]
          tunnel: w369 -> [w380 _]
          tunnel: [w379 w384] -> w367
          tunnel: [w378 w383] -> w368
          tunnel: w365 -> [_ w388]
          frame False {
            n157 = call <vilib>:"IMAQdx Grab2.vi"("Timeout (ms)"=w382, "error in"=w381, "Image In"=w377, "Session In"=w380) -> ("error out"=w379:errorcluster, "Image Out"=w378:T2)  [unwired: 4 in, 2 out]
          }
          frame True {
            n158 = Current VI's Path() -> (path=w389:path)
            n159 = Strip Path(path=w389) -> (stripped path=w390:path)  [unwired: 1 out]
            n160 = Build Path(base path=w390, name or relative path=w388) -> (appended path=w387:path)
            n161 = call "IMAQ ReadFile 2"("File Path"=w387, "error in (no error)"=w385, "Image"=w386) -> ("error out"=w384:errorcluster, "Image Out"=w383:T2)  [unwired: 4 in, 3 out]
          }
        }
        n162 = Bundle By Name(cluster=w374, "Camera data.Image"=w368) -> (w373:T7)
        n163 = call <vilib>:"Add State(s) to Queue__jki_lib_state_machine.vi"("State(s) in (\"\")"=w376) -> ("States Out"=w375:string)  [unwired: 14 in]
      }
      frame "Camera: Add Data" {
        n164 = Unbundle By Name(w419) -> ("Camera data.Image"=w391:T2, "Measurement.Value"=w409:dbl, "Measurement.LinePosY"=w397:i32, "Measurement.Is Alarm On"=w396:bool)
        n165 = call "GetLinePoints.vi"("error in (no error)"=w402, "LinePosY"=w397, "Image"=w391) -> ("error out"=w403:errorcluster, "End Point"=w408:cluster{"X":i32, "Y":i32}, "Start Point"=w412:cluster{"X":i32, "Y":i32})  [unwired: 6 in]
        n166 = call "IMAQ Overlay Line"("Color"=u32 8388608, "error in (no error)"=w403, "End Point"=w408, "Start Point"=w412, "Image"=w391) -> ("error out"=w410:errorcluster, "Image Out"=w413:T2)  [unwired: 5 in]
        n167 = call "GetTextPoint.vi"("End Point"=w408, "Y Offset"=0 ("y"), "X Offset"=-20 ("y")) -> ("Text Point"=w414:cluster{"X":i32, "Y":i32})  [unwired: 8 in]
        n168 = call "TextProperties.vi"("Font Multiplier"=0.05 ("x"), "Image"=w391) -> ("error out"=w398:errorcluster, "Font, Size & Style"=w400:T14)  [unwired: 8 in]
        n169 = Select(t=u32 16711680 ("Text Color (black)"), s=w396, f=u32 0 ("Text Color (black)")) -> (s? t:f=w404:u32)
        n170 = call "FormatPercentage.vi"("Precision"=i16 2 ("precision (6)"), "Raw Percentage"=w409) -> ("Formatted Percentage"=w411:string)  [unwired: 9 in]
        n171 = call "IMAQ Overlay Text"("Text Color (black)"=w404, "Font, Size & Style"=w400, "error in (no error)"=w410, "String"=w411, "Origin"=w414, "Image"=w413) -> ("error out"=w394:errorcluster, "Image Out"=w393:T2)  [unwired: 4 in]
        n172 = call "IMAQ Merge Overlay"("error in (no error)"=w394, "Image Src"=w393) -> ("error out"=w395:errorcluster, "Image Dst Out"=w392:T2)  [unwired: 8 in]
        n173 = Merge Errors(w398, w395) -> (w399:errorcluster)
        n174 = Bundle By Name(cluster=w419, "Camera data.Image"=w392) -> (w418:T7)
        n175 = call <vilib>:"Add State(s) to Queue__jki_lib_state_machine.vi"("State(s) in (\"\")"=w421) -> ("States Out"=w420:string)  [unwired: 14 in]
      }
      frame "Camera: Display" {
        n176 = Unbundle By Name(w422) -> ("Camera data.Image"=→"Image":T2)
        n177 = call <vilib>:"Add State(s) to Queue__jki_lib_state_machine.vi"("State(s) in (\"\")"=w426) -> ("States Out"=w425:string)  [unwired: 14 in]
      }
      frame "Camera: Remove" {
        n178 = Unbundle By Name(w430) -> ("Camera data.Camera"=w429:T1)
        n179 = call <vilib>:"IMAQdx Close Camera.vi"("error in"=w428, "Session In"=w429) -> ("error out"=w427:errorcluster)  [unwired: 9 in]
        n180 = call <vilib>:"Add State(s) to Queue__jki_lib_state_machine.vi"("State(s) in (\"\")"=w432) -> ("States Out"=w431:string)  [unwired: 14 in]
      }
      frame "---------- Python ----------" {
        # "Do not put any code in this frame.\n(It is a separator no-op. You can make a copy of this frame to create a new Macro frame)"
        n181 = call <vilib>:"Add State(s) to Queue__jki_lib_state_machine.vi"("State(s) in (\"\")"=w436) -> ("States Out"=w435:string)  [unwired: 14 in]
      }
      frame "Python: Open Session" {
        n182 = Unbundle By Name(w439) -> ("Python info.Python version"=w442:string)
        n183 = Open Python Session(python version=w442, 3:w441) -> (session out=w438:refnum<k35>, error out=w440:errorcluster)  [unwired: 1 in]
        n184 = Bundle By Name(cluster=w439, "Python info.Session reference"=w438) -> (w437:T7)
        n185 = call <vilib>:"Add State(s) to Queue__jki_lib_state_machine.vi"("State(s) in (\"\")"=w444) -> ("States Out"=w443:string)  [unwired: 14 in]
      }
      frame "Python: Fetch Level" {
        # "If there's no error, the status is false, therefore we can say the measurement is done."
        n186 = Unbundle By Name(w456) -> ("Python info.Session reference"=w463:refnum<k35>, "Python info.Module name"=w460:string, "Python info.Function name"=w458:string, "Camera data.Use image"=w450:bool, "Camera data.Image name"=w449:string)
        n187 = Current VI's Path() -> (path=w462:path)
        n188 = Strip Path(path=w462) -> (stripped path=w461:path)  [unwired: 1 out]
        n189 = Build Path(base path=w461, name or relative path=w460) -> (appended path=w459:path)
        n190 = node(w463, w459, w458, w464, cluster{"Value":dbl, "LinePosY":i32} {"Value"=0.0, "LinePosY"=0}, w450, w449) -> (w452:errorcluster, w447:cluster{"Value":dbl, "LinePosY":i32})  [unwired: 2 in, 3 out]
        n191 = Get Date/Time In Seconds() -> (seconds since 1Jan1904=w457:timestamp)
        n192 = Unbundle By Name(w447) -> ("Value"=w445:dbl, "LinePosY"=w446:i32)
        "Measurement" <- w445
        n193 = call-poly <vilib>:"DB Tools Format Datetime String.vi"("time stamp"=w457) -> ("date/time string"=w454:string)
        n194 = Bundle By Name(cluster=w456, "Measurement.Date"=w454, "Measurement.Value"=w445, "Measurement.LinePosY"=w446) -> (w455:T7)
        n195 = Unbundle By Name(w452) -> ("status"=w451:bool)
        n196 = property on="Measuring" class="Bool (strict)"("Value"=w451) -> ()  [unwired: 2 in, 2 out]
        n197 = call <vilib>:"Add State(s) to Queue__jki_lib_state_machine.vi"("State(s) in (\"\")"=w466) -> ("States Out"=w465:string)  [unwired: 14 in]
        "Measuring" <- TRUE ("Measuring")
      }
      frame "Python: Close Session" {
        n198 = Unbundle By Name(w468) -> ("Python info.Session reference"=w467:refnum<k35>)
        n199 = Close Python Session(session in=w467, error in=w470) -> (11:w469:errorcluster)
        n200 = call <vilib>:"Add State(s) to Queue__jki_lib_state_machine.vi"("State(s) in (\"\")"=w472) -> ("States Out"=w471:string)  [unwired: 14 in]
      }
      frame "---------- Safety ----------" {
        # "Do not put any code in this frame.\n(It is a separator no-op. You can make a copy of this frame to create a new Macro frame)"
        n201 = call <vilib>:"Add State(s) to Queue__jki_lib_state_machine.vi"("State(s) in (\"\")"=w476) -> ("States Out"=w475:string)  [unwired: 14 in]
      }
      frame "Safety: Error Cleanup" {
        # "Blindly close sessions and connections regardless of whether they're open or not. In case errors are raised, ignore them in Error Handler state."
        n202 = Bundle By Name(cluster=w480, "Measurement.Is On"=FALSE) -> (w478:T7)
        n203 = property on="Error" class="Bool (strict)"("Blinking"=TRUE) -> ()  [unwired: 2 in, 2 out]
        n204 = property on="Is Measurement On" class="Bool (strict)"("Value"=FALSE ("Is Measurement On")) -> ()  [unwired: 2 in, 2 out]
        n205 = call <vilib>:"Add State(s) to Queue__jki_lib_state_machine.vi"("State(s) in Front (\"\")"="Macro: Stop Measurement" ("State(s) in Front (\"\")"), "State(s) in (\"\")"=w485) -> ("States Out"=w484:string)  [unwired: 13 in]
      }
      frame "Safety: Check Alarm Level" {
        n206 = Unbundle By Name(w488) -> ("Measurement.Value"=w491:dbl, "Measurement.Threshold"=w490:dbl)
        n207 = Greater?(x=w491, y=w490) -> (0:w486:bool)
        n208 = Bundle By Name(cluster=w488, "Measurement.Is Alarm On"=w486) -> (w487:T7)
        n209 = property on="Alarm" class="Bool (strict)"("Blinking"=w486) -> ()  [unwired: 2 in, 2 out]
        n210 = call <vilib>:"Add State(s) to Queue__jki_lib_state_machine.vi"("State(s) in (\"\")"=w493) -> ("States Out"=w492:string)  [unwired: 14 in]
      }
    }
  }
